vi "updateColoursInBackground.vi"(8 "error in (no error)":errorcluster, 11 "ScriptEditorV2 in":refnum<class "ScriptEditorV2.lvclass">) -> (0 "error out":errorcluster, 3 "ScriptEditorV2 out":refnum<class "ScriptEditorV2.lvclass">)   [LabVIEW 2011, in "Views.lvlib" / "ScriptEditor.lvlib" / "ScriptEditorV2.lvclass"]
uses:
  ScriptEditorV2.lvclass
  Tools/Filing/FileSystem/FileSystem.lvclass
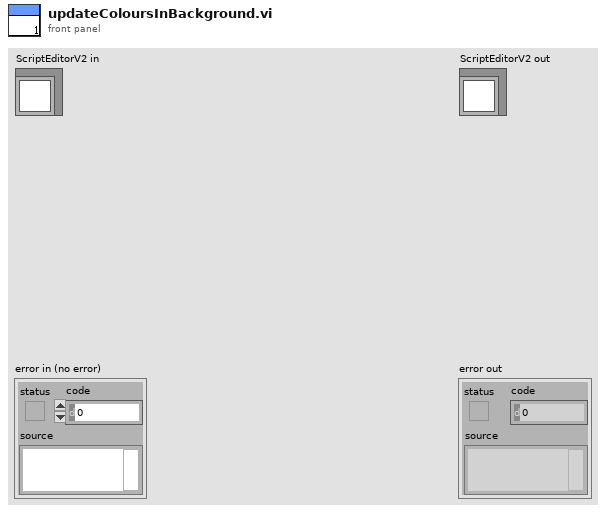
[diagram p1: front panel]
types:
  T1 = enum32{"Bad", "Idle", "Run top level", "Running"}
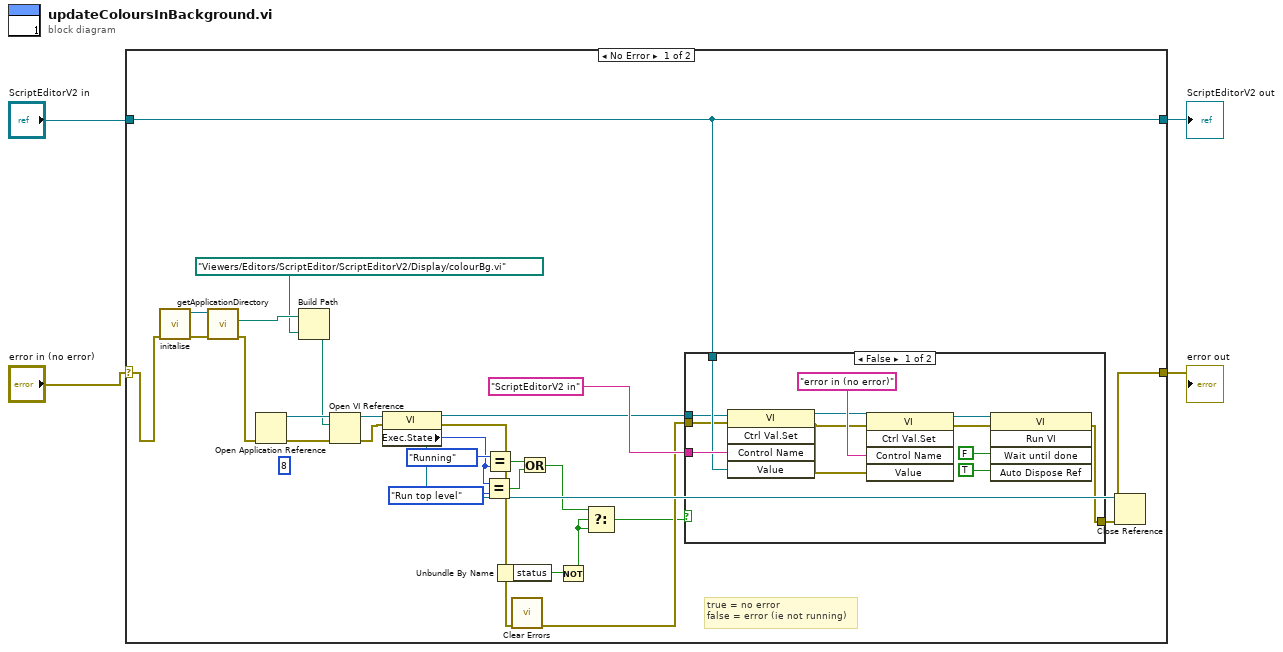
[diagram p0: block diagram]
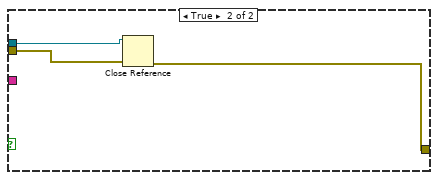
[diagram p2: hidden frame]
diagram:
  n1 = case shown="No Error" "error in (no error)" {
    selector: "error in (no error)" -> [w22 w48]
    tunnel: [w28 w48] -> w1
    tunnel: "ScriptEditorV2 in" -> [w19 w47]
    tunnel: [w19 w47] -> w2
    frame No Error {
      (unwired) 8 ("options")
      # "true = no error\nfalse = error (ie not running)"
      n2 = call "initalise.vi"("error in (no error)"=w22) -> ("error out"=w24:errorcluster, "FileSystem out"=w23:refnum<class "FileSystem.lvclass">)  [unwired: 9 in]
      n3 = call-dynamic "getApplicationDirectory.vi"("error in (no error)"=w24, "FileSystem.lvclass in"=w23) -> ("error out"=w21:errorcluster, "ApplicationDirectory"=w26:path)  [unwired: 7 in, 1 out]
      n4 = Open Application Reference(8:w21) -> (0:w31:errorcluster, 3:w30:refnum<vi>)  [unwired: 3 in]
      n5 = Build Path(base path=w26, name or relative path=path "Viewers/Editors/ScriptEditor/ScriptEditorV2/Display/colourBg.vi" ("vi path")) -> (appended path=w20:path)
      n6 = Open VI Reference(application reference (local)=w30, vi path=w20, error in (no error)=w31) -> (vi reference=w18:refnum<vi>, error out=w12:errorcluster)  [unwired: 3 in]
      n7 = property class="VI"(reference=w18, error in=w12) -> (reference out=w17:refnum<vi>, error out=w7:errorcluster, "Exec.State"=w11:T1)
      n8 = Equal?(x=w11, y=T1."Run top level" ("Execution:State")) -> (x = y?=w13:bool)
      n9 = Equal?(x=T1."Running" ("Execution:State"), y=w11) -> (x = y?=w14:bool)
      n10 = Unbundle By Name(w7) -> ("status"=w10:bool)
      n11 = call <vilib>:"Clear Errors.vi"("error in (no error)"=w7) -> ("error out"=w6:errorcluster)  [unwired: 6 in]
      n12 = Or(x=w14, y=w13) -> (x .or. y?=w8:bool)
      n13 = Not(x=w10) -> (.not. x?=w9:bool)
      n14 = Select(t=w8, s=w9, f=w9) -> (s? t:f=w5:bool)
      n15 = case shown="False" w5 {
        tunnel: [w38 w44] -> w29
        tunnel: "ScriptEditorV2 in" ("Control Name") -> [w35 _]
        tunnel: w19 -> [w34 _]
        tunnel: w17 -> [w33 w46]
        tunnel: w6 -> [w32 w45]
        frame False {
          n16 = invoke class="VI" method="Ctrl Val.Set"(reference=w33, error in=w32, "Control Name"=w35, "Value"=w34) -> (reference out=w40:refnum<vi>, error out=w39:errorcluster)  [unwired: 1 in, 3 out]
          n17 = invoke class="VI" method="Ctrl Val.Set"(reference=w40, error in=w39, "Control Name"="error in (no error)", "Value"=w39) -> (reference out=w37:refnum<vi>, error out=w36:errorcluster)  [unwired: 1 in, 3 out]
          n18 = invoke class="VI" method="Run VI"(reference=w37, error in=w36, "Wait until done"=FALSE, "Auto Dispose Ref"=TRUE) -> (error out=w38:errorcluster)  [unwired: 1 in, 4 out]
        }
        frame True {
          n19 = Close Reference(reference=w46, error in (no error)=w45) -> (error out=w44:errorcluster)
        }
      }
      n20 = Close Reference(reference=w30, error in (no error)=w29) -> (error out=w28:errorcluster)
    }
    frame Error {
    }
  }
  "error out" <- w1
  "ScriptEditorV2 out" <- w2
